vi "Read DefaultPythonVersion.vi"(8 "error in (no error)":errorcluster, 11 "ArgparseWrapper in":refnum<class "ArgparseWrapper.lvclass">) -> (0 "error out":errorcluster, 2 "DefaultPythonVersion":string="3.9", 3 "ArgparseWrapper out":refnum<class "ArgparseWrapper.lvclass">)   [LabVIEW 2022 SP3, in "ArgumentParser.lvlib" / "ArgparseWrapper.lvclass"]
uses:
  ArgparseWrapper.lvclass
  ArgparseWrapper.lvclass/ArgparseWrapper.ctl
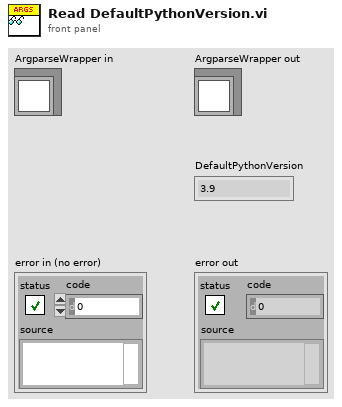
[diagram p1: front panel]
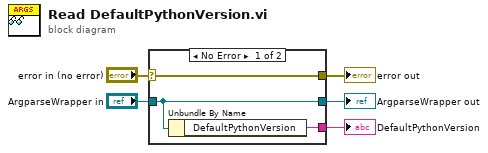
[diagram p0: block diagram]
diagram:
  n1 = case shown="No Error" "error in (no error)" {
    selector: "error in (no error)" -> [w8 w9]
    tunnel: [w8 w9] -> w4
    tunnel: [w7 w10] -> w2
    tunnel: "ArgparseWrapper in" -> [w7 w10]
    tunnel: [w6 _] -> w1
    frame No Error {
      n2 = Unbundle By Name(w7) -> ("DefaultPythonVersion"=w6:string)
    }
    frame Error {
    }
  }
  "error out" <- w4
  "ArgparseWrapper out" <- w2
  "DefaultPythonVersion" <- w1
